vi "add channel to configuration.vi"(8 "error in":errorcluster, 10 "channel":refnum<class "TBM channel.lvclass">, 11 "alarms module configuration in":refnum<class "alarms module configuration.lvclass">) -> (0 "error out":errorcluster, 3 "alarms module configuration out":refnum<class "alarms module configuration.lvclass">)   [LabVIEW 2013, in "alarms module configuration.lvclass"]
uses:
  alarms module configuration.lvclass
  <vilib>/NI/Tag Bus/tag/tag descriptor.lvclass
  <vilib>/NI/Tag Bus Module Framework/channel/TBM channel.lvclass
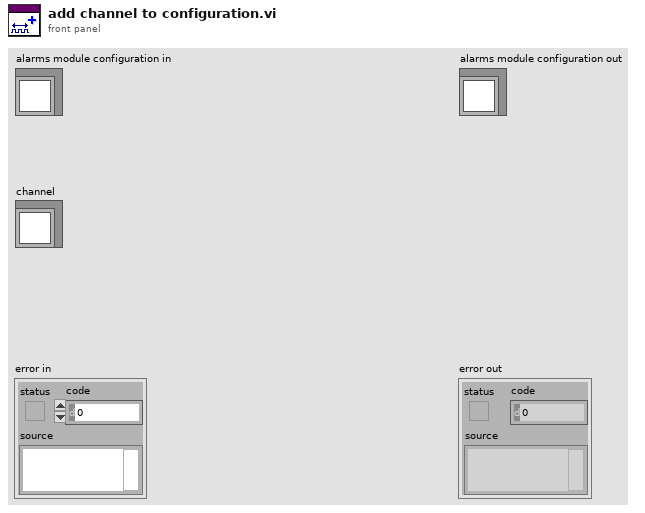
[diagram p1: front panel]
types:
  T1 = typedef "alarms module configuration.lvclass/alarm configuration.ctl" = cluster{"comparison":string, "comparisons":T2[], "unlatch":refnum<class "TBM channel.lvclass">, "output":refnum<class "TBM channel.lvclass">, "boolean op":T4}
  T2 = typedef "alarms module configuration.lvclass/alarm comparison.ctl" = cluster{"input channel":refnum<class "TBM channel.lvclass">, "limit":dbl, "comparison":T3}
  T3 = typedef "alarms module configuration.lvclass/compare type.ctl" = enum16{">", "<", ">=", "<=", "="}
  T4 = typedef "alarms module configuration.lvclass/boolean operation.ctl" = enum16{"AND", "OR"}
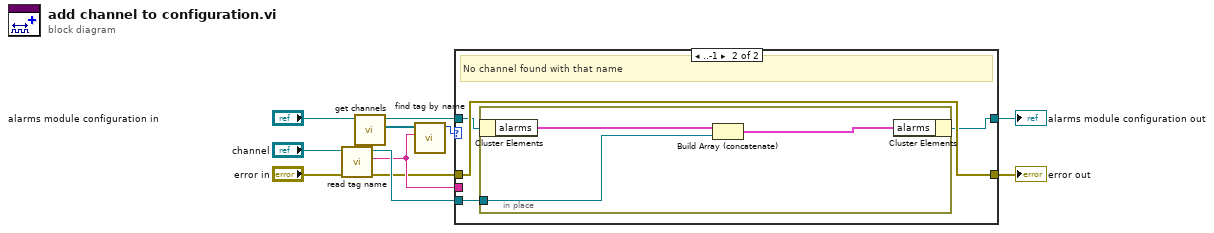
[diagram p0: block diagram]
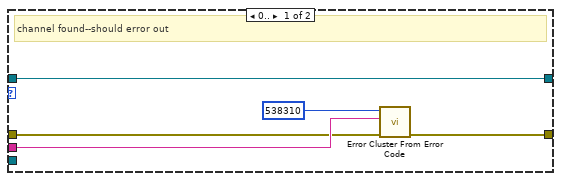
[diagram p2: hidden frame]
diagram:
  n1 = call <vilib>:"read tag name.vi"("error in"="error in", "system tag in"="channel") -> ("error out"=w2:errorcluster, "name"=w3:string, "system tag out"=w10:refnum<class "TBM channel.lvclass">)  [unwired: 7 in]
  n2 = call-dynamic "get channels.vi"("alarms module configuration in"="alarms module configuration in") -> ("channels"=w5:refnum<class "TBM channel.lvclass">[], "alarms module configuration out"=w11:refnum<class "alarms module configuration.lvclass">)  [unwired: 9 in]
  n3 = call <vilib>:"find tag by name.vi"("name"=w3, "tags in"=w5) -> ("index"=w4:i32)  [unwired: 9 in]
  n4 = case shown="..-1" w4 {
    tunnel: [w16 w19] -> w8
    tunnel: w3 -> [w14 _]
    tunnel: w2 -> [w13 w19]
    tunnel: w11 -> [w12 w18]
    tunnel: w10 -> [_ w20]
    tunnel: [w12 w17] -> w7
    frame 0.. {
      # "channel found--should error out"
      n5 = call <vilib>:"Error Cluster From Error Code.vi"("error in (no error)"=w13, "error message (\"\")"=w14, "error code (0)"=538310) -> ("error out"=w16:errorcluster)  [unwired: 6 in]
    }
    frame ..-1 {
      # "No channel found with that name"
      n6 = in-place {
        in-place-border: w20 -> [w23]
        n7 = in-place-cluster #1(w18) -> ("alarms"=w21:T1[])
        n8 = Build Array (concatenate)(w21, w23) -> (w22:T1[])
        n9 = in-place-cluster #1("alarms"=w22) -> (w17:refnum<class "alarms module configuration.lvclass">)
      }
    }
  }
  "error out" <- w8
  "alarms module configuration out" <- w7
